vi "resetProfileStepCounter.vi"(8 "error in (no error)":errorcluster, 11 "Model in":refnum<class "Model.lvclass">) -> (0 "error out":errorcluster, 3 "Model out":refnum<class "Model.lvclass">)   [LabVIEW 2013, in "Model.lvclass"]
uses:
  Model.lvclass
  Model.lvclass/Model.ctl
  ApplicationElements/Logger/Logger.lvclass/Logger.ctl
  ApplicationElements/TestMonitor/TestMonitor.lvclass
  ApplicationElements/Logger/Logger.lvclass
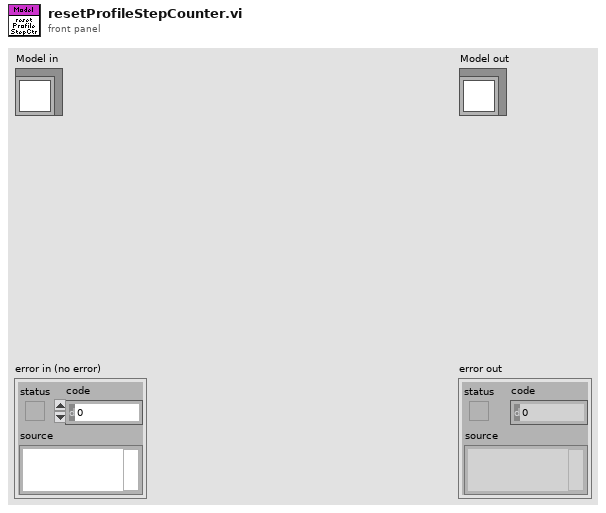
[diagram p1: front panel]
types:
  T1 = typedef "M2AADTTypedefs.lvlib/TestStatus.ctl" = cluster{"activeCycle":u32, "activeProfileStep":u32}
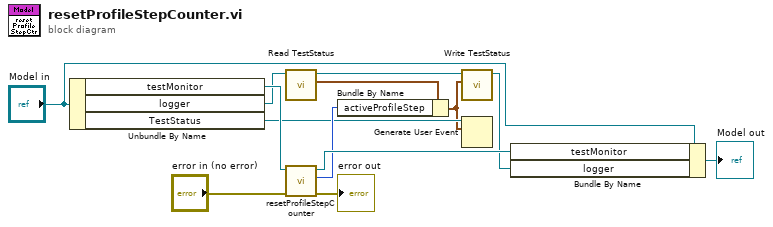
[diagram p0: block diagram]
diagram:
  n1 = Unbundle By Name("Model in") -> ("testMonitor"=w13:refnum<class "TestMonitor.lvclass">, "logger"=w6:refnum<class "Logger.lvclass">, "TestStatus"=w2:refnum<user-event>)
  n2 = call "Read TestStatus.vi"("Logger in"=w6) -> ("TestStatus"=w7:T1, "Logger out"=w5:refnum<class "Logger.lvclass">)  [unwired: 9 in]
  n3 = call "resetProfileStepCounter.vi"("error in (no error)"="error in (no error)", "TestMonitor in"=w13) -> ("error out"=→"error out":errorcluster, "activeProfileStep"=w3:u32, "TestMonitor out"=w8:refnum<class "TestMonitor.lvclass">)  [unwired: 7 in]
  n4 = Bundle By Name(cluster=w7, "activeProfileStep"=w3) -> (w1:T1)
  n5 = call "Write TestStatus.vi"("TestStatus"=w1, "Logger in"=w5) -> ("Logger out"=w4:refnum<class "Logger.lvclass">)  [unwired: 9 in]
  n6 = Generate User Event(user event=w2, event data cluster=w1) -> ()  [unwired: 2 in, 2 out]
  n7 = Bundle By Name(cluster="Model in", "testMonitor"=w8, "logger"=w4) -> (→"Model out":refnum<class "Model.lvclass">)
